vi "Helper SubVI - Subroutine.vi"(10 "Numeric In":dbl) -> (2 "Numeric Out":dbl)   [LabVIEW 2023]
doc: "This VI runs at subroutine priority. A subroutine VI gains control of its owning thread when running. This results in the best possible performance of the VI, at the expense of any other VIs running in the same thread."
panel:
  # "This VI is set to subroutine priority in its execution properties."
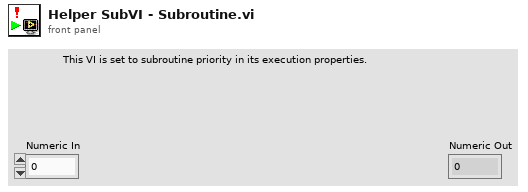
[diagram p1: front panel]
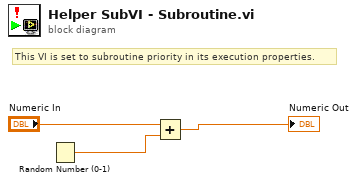
[diagram p0: block diagram]
diagram:
  # "This VI is set to subroutine priority in its execution properties."
  n1 = Random Number (0-1)() -> (number: 0 to 1=w1:dbl)
  n2 = Add(x="Numeric In", y=w1) -> (x+y=→"Numeric Out":dbl)
